vi "Hide Edit Controls if Scrolled.vi"(11 "Settings UI in":refnum<class "Settings UI.lvclass">) -> (3 "Settings UI out":refnum<class "Settings UI.lvclass">)   [LabVIEW 2020, in "Output Sequencer.lvlib" / "Settings UI.lvclass"]
uses:
  Settings UI.lvclass
  Settings UI.lvclass/Settings UI.ctl
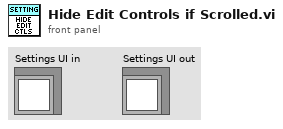
[diagram p1: front panel]
types:
  T1 = typedef "LVNodeAndColumnTypeDef.ctl" = cluster{"Node":string, "Column":i32}
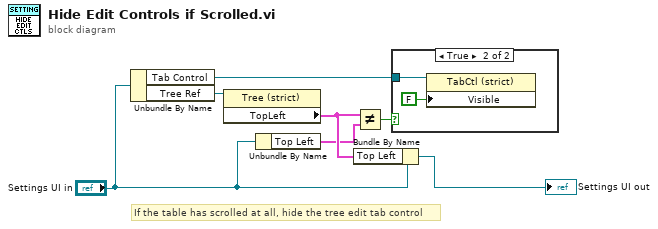
[diagram p0: block diagram]
diagram:
  # "If the table has scrolled at all, hide the tree edit tab control"
  n1 = Unbundle By Name("Settings UI in") -> ("Tab Control"=w5:refnum<vi>, "Tree Ref"=w2:refnum<vi>)
  n2 = property class="Tree (strict)"(reference=w2) -> ("TopLeft"=w4:T1)  [unwired: 1 in, 2 out]
  n3 = Unbundle By Name("Settings UI in") -> ("Top Left"=w3:T1)
  n4 = Bundle By Name(cluster="Settings UI in", "Top Left"=w4) -> (→"Settings UI out":refnum<class "Settings UI.lvclass">)
  n5 = Not Equal?(x=w4, y=w3) -> (x != y?=w6:bool)
  n6 = case shown="True" w6 {
    tunnel: w5 -> [_ w8]
    frame False {
    }
    frame True {
      n7 = property on="Property Node" class="TabCtl (strict)"(reference=w8, "Visible"=FALSE) -> ()  [unwired: 1 in, 2 out]
    }
  }
